vi "Test.Maui 2.0.Ring Value Change.vi"(8 "error in":errorcluster) -> (0 "error out":errorcluster)   [LabVIEW 2020]
uses:
  Maui 2.0/Maui 2.0.lvclass
  C:/Program Files (x86)/National Instruments/LabVIEW 2020/vi.lib/JKI/JKI SMO/SMO/SMO.lvclass
  Helper/Test Helper 1/Test Helper 1.lvclass
  <vilib>/addons/_JKI Toolkits/Caraya/classes/Assert/Assert Equal Value_Variant.vi
  <vilib>/JKI/JKI SMO/SMO/SMO.lvclass
  <vilib>/addons/_JKI Toolkits/Caraya/classes/Test/Test.lvclass
  <vilib>/addons/_JKI Toolkits/Caraya/classes/Assert/Assert.lvclass
panel:
  in  "Ring 2":u16(ring) items=["Test Helper 1", "Test Helper 1", "Test Helper 1", "None"]
  in  "Ring":u16(ring) items=["Test Helper 1", "Test Helper 1", "Test Helper 1", "None"]
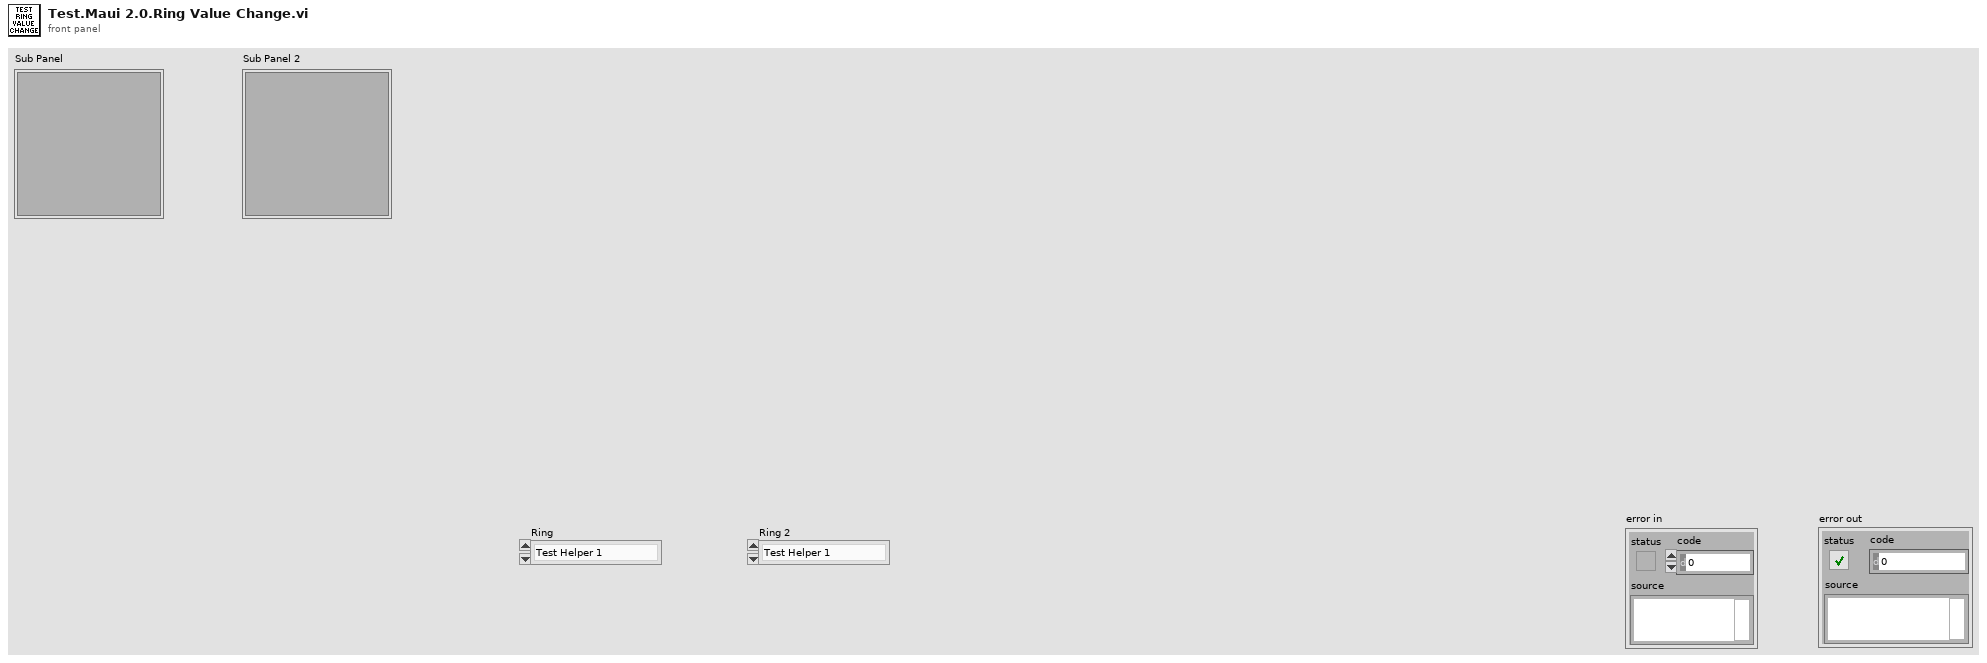
[diagram p1: front panel]
types:
  T1 = cluster{"Ring":refnum<vi>, "Sub Panel":refnum<vi>}
  T2 = cluster{"Ring 2":refnum<vi>, "Sub Panel 2":refnum<vi>}
  T3 = cluster{"Ring 2":refnum<vi>, "Sub Panel 2":refnum<vi>}[]
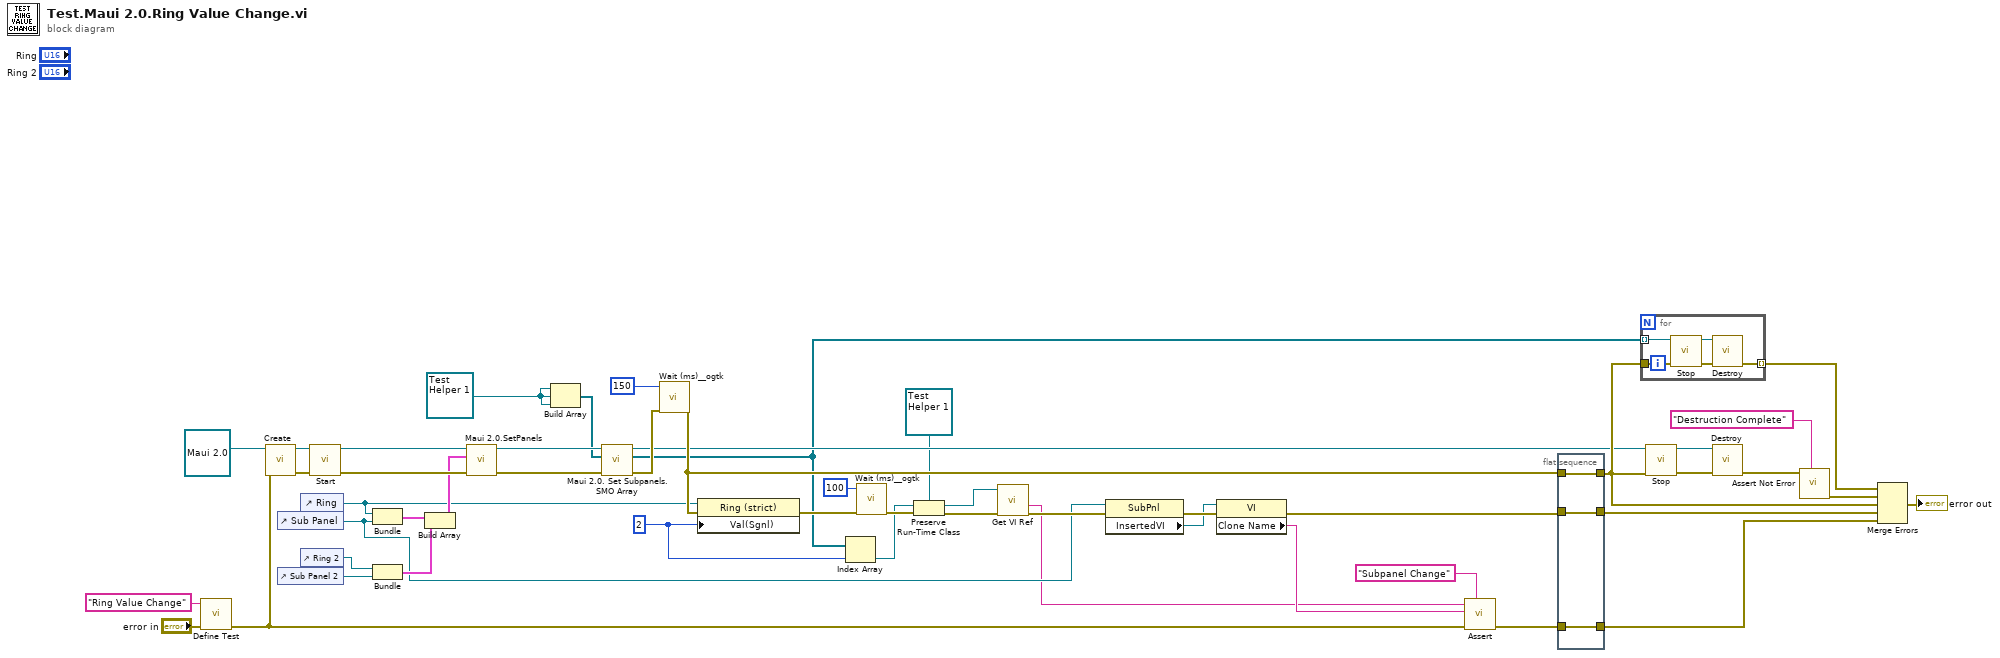
[diagram p0: block diagram]
diagram:
  w9 = u16 2 ("Value (Signaling)")
  w11 = refnum<class "Test Helper 1.lvclass"> refnum ("Test Helper 1.lvclass")
  n1 = call <vilib>:"Define Test.vi"("error in (no error)"="error in", "Label (VI Title)"="Ring Value Change") -> ("error out"=w40:errorcluster)  [unwired: 9 in]
  n2 = call <vilib>:"Create.vi"("error in (no error)"=w40, "SMO"=refnum<class "Maui 2.0.lvclass"> refnum ("Maui 2.0 in")) -> ("error out"=w50:errorcluster, "SMO out"=w25:refnum<class "Maui 2.0.lvclass">)  [unwired: 7 in, 1 out]
  n3 = control-ref of="Sub Panel"() -> (w5:refnum<vi>)
  n4 = control-ref of="Sub Panel 2"() -> (w28:refnum<vi>)
  n5 = control-ref of="Ring"() -> (w12:refnum<vi>)
  n6 = control-ref of="Ring 2"() -> (w29:refnum<vi>)
  n7 = call <vilib>:"Start.vi"("error in (no error)"=w50, "SMO"=w25) -> ("error out"=w49:errorcluster, "SMO out"=w23:refnum<class "Maui 2.0.lvclass">)  [unwired: 8 in]
  n8 = Bundle("Ring"=w12, "Sub Panel"=w5) -> (w27:T1)  [unwired: 1 in]
  n9 = Bundle("Ring 2"=w29, "Sub Panel 2"=w28) -> (w26:T2)  [unwired: 1 in]
  n10 = Build Array(w27, w26) -> (w20:T3)
  n11 = call "Maui 2.0.SetPanels.vi"("error in (no error)"=w49, "Set Panels"=w20, "Maui 2.0"=w23) -> ("error out"=w48:errorcluster, "Maui 2.0 out"=w22:refnum<class "Maui 2.0.lvclass">)  [unwired: 7 in]
  n12 = Build Array(w11, w11, w11) -> (w21:refnum<class "Test Helper 1.lvclass">[])
  n13 = call-dynamic "Maui 2.0. Set Subpanels.SMO Array.vi"("error in (no error)"=w48, "Subpanels in"=w21, "Maui 2.0 in"=w22) -> ("error out"=w42:errorcluster, "Subpanels Out"=w10:refnum<class "SMO.lvclass">[], "Maui 2.0 out"=w17:refnum<class "Maui 2.0.lvclass">)  [unwired: 6 in]
  n14 = call <userlib>:"Wait (ms)__ogtk.vi"("error in (no error)"=w42, "milliseconds to wait"=u32 150) -> ("error out"=w36:errorcluster)  [unwired: 8 in, 1 out]
  n15 = property on="Property Node" class="Ring (strict)"(reference=w12, error in=w36, "Val(Sgnl)"=w9) -> (error out=w31:errorcluster)  [unwired: 1 out]
  n16 = Index Array(array=w10, index=w9) -> (element=w8:refnum<class "SMO.lvclass">)
  n17 = call <userlib>:"Wait (ms)__ogtk.vi"("error in (no error)"=w31, "milliseconds to wait"=u32 100) -> ("error out"=w30:errorcluster)  [unwired: 8 in, 1 out]
  n18 = Preserve Run-Time Class(object in=w8, error in=w30, 2:refnum<class "Test Helper 1.lvclass"> refnum ("Test Helper 1.lvclass")) -> (object out=w4:refnum<class "Test Helper 1.lvclass">, error out=w33:errorcluster)
  n19 = call-dynamic "Get VI Ref.vi"("error in (no error)"=w33, "Test Helper 1 in"=w4) -> ("error out"=w35:errorcluster, "VI Clone Name"=w2:string)  [unwired: 6 in, 2 out]
  n20 = property on="Property Node" class="SubPnl"(reference=w5, error in=w35) -> (error out=w34:errorcluster, "InsertedVI"=w6:refnum<vi>)  [unwired: 1 out]
  n21 = property on="Property Node" class="VI"(reference=w6, error in=w34) -> (error out=w32:errorcluster, "Clone Name"=w3:string)  [unwired: 1 out]
  n22 = call-poly <vilib>:"Assert.vi"("Label"="Subpanel Change", "error in (no error)"=w40, "Y"=w3, "X"=w2) -> ("error out"=w39:errorcluster)  [unwired: 7 in]
  n23 = flat-sequence {
    tunnel: w36 -> [w53]
    tunnel: w32 -> [w52]
    tunnel: w39 -> [w51]
    tunnel: [w53] -> w41
    tunnel: [w52] -> w44
    tunnel: [w51] -> w43
    frame #0 {
    }
  }
  n24 = for {
    tunnel: w10 -> [w54] mode=indexing
    tunnel: w41 -> [w58]
    tunnel: [w56] -> w14 mode=indexing
    n25 = call <vilib>:"Stop.vi"("error in (no error)"=w58, "SMO"=w54) -> ("error out"=w57:errorcluster, "SMO out"=w55:refnum<class "SMO.lvclass">)  [unwired: 8 in]
    n26 = call <vilib>:"Destroy.vi"("error in (no error)"=w57, "SMO"=w55) -> ("error out"=w56:errorcluster)  [unwired: 9 in]
  }
  n27 = call <vilib>:"Stop.vi"("error in (no error)"=w41, "SMO"=w17) -> ("error out"=w47:errorcluster, "SMO out"=w16:refnum<class "Maui 2.0.lvclass">)  [unwired: 8 in]
  n28 = call <vilib>:"Destroy.vi"("error in (no error)"=w47, "SMO"=w16) -> ("error out"=w46:errorcluster)  [unwired: 9 in]
  n29 = call <vilib>:"Assert Not Error.vi"("Label"="Destruction Complete", "Not Error?"=w46) -> ("error out"=w45:errorcluster)  [unwired: 9 in]
  n30 = Merge Errors(w14, w45, w41, w44, w43) -> (→"error out":errorcluster)
